vi "Read Sensor Data.vi"(8 "error in (no error)":errorcluster, 10 "wait ms":u32=500, 11 "VISA Refnum in":refnum<visa-resource-name>) -> (0 "error out":errorcluster, 1 "DataOut":T1, 2 "read buffer":string, 3 "VISA Refnum out":refnum<visa-resource-name>, 5 "Data Not Good":bool)   [LabVIEW 2013]
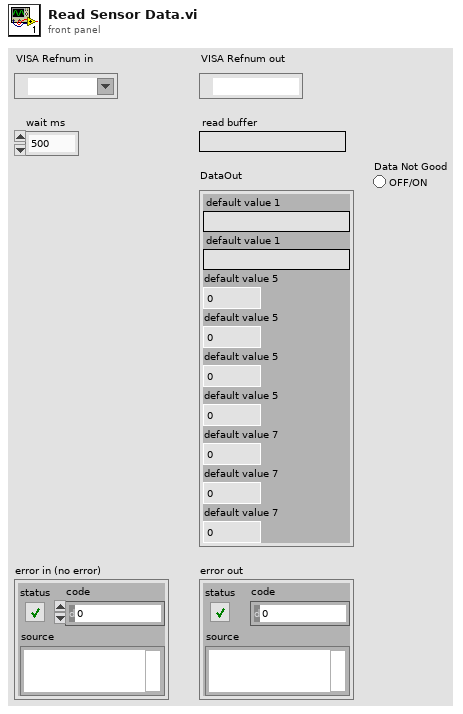
[diagram p1: front panel]
types:
  T1 = cluster{"default value 1":string, "default value 1":string, "default value 5":u32, "default value 5":u32, "default value 5":u32, "default value 5":u32, "default value 7":sgl, "default value 7":sgl, "default value 7":sgl}
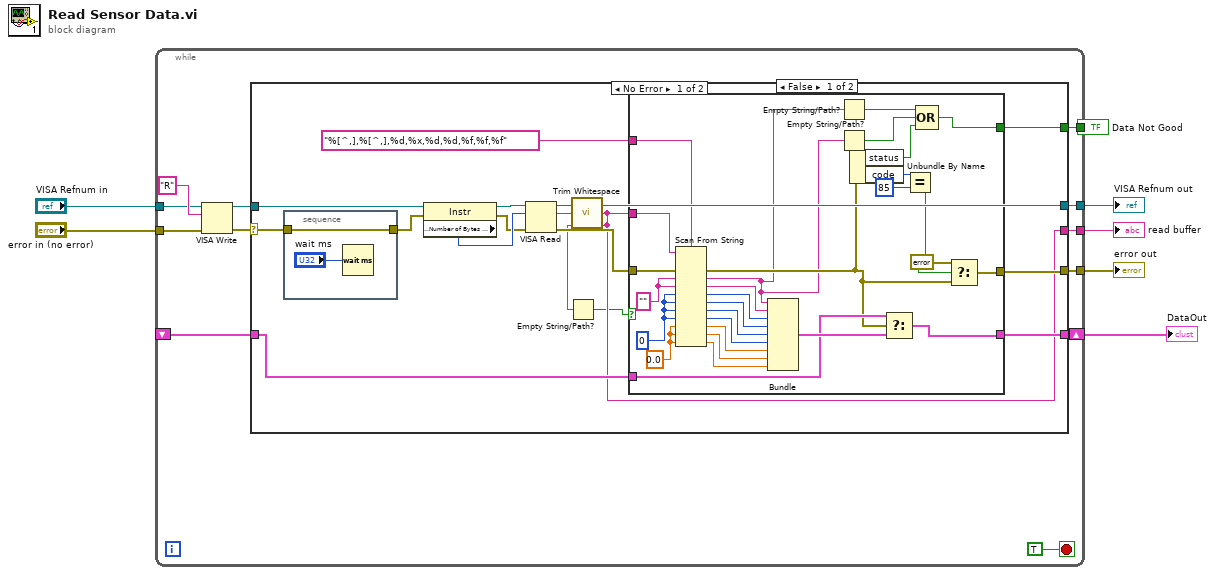
[diagram p0: block diagram]
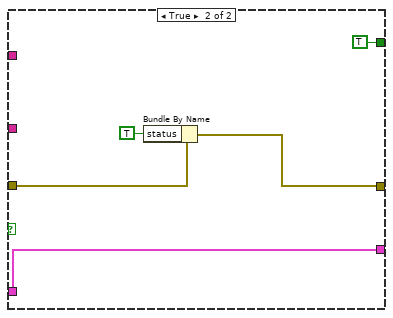
[diagram p2: hidden frame]
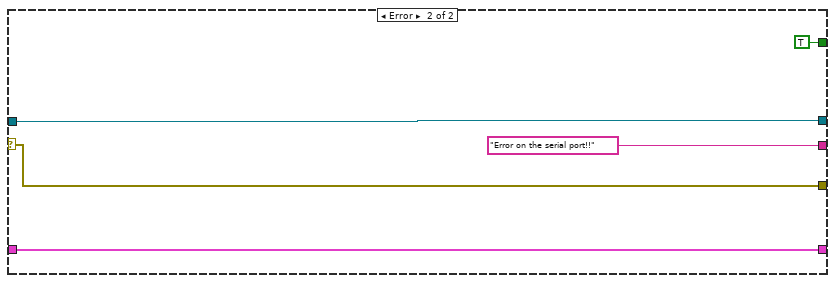
[diagram p3: hidden frame]
diagram:
  n1 = while {
    tunnel: "error in (no error)" -> [w16]
    tunnel: "VISA Refnum in" -> [w15]
    tunnel: [w13] -> w4
    tunnel: [w12] -> w3
    tunnel: [w11] -> w2
    tunnel: [w9] -> w1
    shift-right: [w14] -> w5
    shift-left: _ -> [w10]
    stop <- TRUE stop-if-true
    n2 = VISA Write(VISA resource name=w15, write buffer="R" ("string"), error in (no error)=w16) -> (VISA resource name out=w17:refnum<visa-resource-name>, error out=w18:errorcluster)  [unwired: 1 out]
    n3 = case shown="No Error" w18 {
      selector: w18 -> [w28 w72]
      tunnel: w17 -> [w30 w75]
      tunnel: [w27 w75] -> w11
      tunnel: [w23 w72] -> w12
      tunnel: [w24 w74] -> w14
      tunnel: [w21 "Error on the serial port!!" ("read buffer")] -> w13
      tunnel: w10 -> [w25 w74]
      tunnel: [w22 TRUE] -> w9
      frame No Error {
        n4 = stacked-sequence {
          tunnel: [w69] -> w31
          tunnel: w28 -> [w69]
          frame #0 {
            n5 = Wait (ms)(milliseconds to wait="wait ms") -> ()  [unwired: 1 out]
          }
        }
        n6 = property class="Instr"(reference=w30, error in=w31) -> (reference out=w33:refnum<visa-resource-name>, error out=w32:errorcluster, "Serial Settings:Number of Bytes at Serial Port"=w34:u32)
        n7 = VISA Read(VISA resource name=w33, byte count=w34, error in (no error)=w32) -> (VISA resource name out=w27:refnum<visa-resource-name>, read buffer=w26:string, error out=w29:errorcluster)  [unwired: 1 out]
        n8 = call <vilib>:"Trim Whitespace.vi"("string"=w26) -> ("trimmed string"=w21:string)  [unwired: 1 in]
        n9 = Empty String/Path?(string/path=w21) -> (empty?=w20:bool)
        n10 = case shown="False" w20 {
          tunnel: "%[^,],%[^,],%d,%x,%d,%d,%f,%f,%f" ("String") -> [w63 _]
          tunnel: w29 -> [w51 w65]
          tunnel: w21 -> [w50 _]
          tunnel: w25 -> [w48 w68]
          tunnel: [w47 w68] -> w24
          tunnel: [w41 w64] -> w23
          tunnel: [w36 TRUE] -> w22
          frame False {
            w53 = sgl 0.0 ("default value 7")
            w62 = "" ("default value 1")
            w52 = u32 0 ("default value 5")
            n11 = Scan From String(format string=w63, input string=w50, error in=w51, default 1=w62, default 2=w62, default 3=w52, default 4=w52, default 5=w52, default 6=w52, default 7=w53, default 8=w53, default 9=w53) -> (error out=w43:errorcluster, output 1=w40:string, output 2=w61:string, output 3=w60:u32, output 4=w59:u32, output 5=w58:u32, output 6=w57:u32, output 7=w56:sgl, output 8=w55:sgl, output 9=w54:sgl)  [unwired: 1 in, 2 out]
            n12 = Bundle("default value 1"=w40, "default value 1"=w61, "default value 5"=w60, "default value 5"=w59, "default value 5"=w58, "default value 5"=w57, "default value 7"=w56, "default value 7"=w55, "default value 7"=w54) -> (w49:T1)  [unwired: 1 in]
            n13 = Empty String/Path?(string/path=w40) -> (empty?=w39:bool)
            n14 = Empty String/Path?(string/path=w40) -> (empty?=w38:bool)
            n15 = Unbundle By Name(w43) -> ("status"=w37:bool, "code"=w46:i32)
            n16 = Select(t=w48, s=w43, f=w49) -> (s? t:f=w47:T1)
            n17 = Equal?(x=w46, y=85) -> (x = y?=w44:bool)
            n18 = Compound Arithmetic op=OR(w39, w38, w37) -> (w36:bool)
            n19 = Select(t=errorcluster {"status"=FALSE, "code"=0, "source"=""}, s=w44, f=w43) -> (s? t:f=w41:errorcluster)
          }
          frame True {
            n20 = Bundle By Name(cluster=w65, "status"=TRUE) -> (w64:errorcluster)
          }
        }
      }
      frame Error {
      }
    }
  }
  "DataOut" <- w5
  "read buffer" <- w4
  "error out" <- w3
  "VISA Refnum out" <- w2
  "Data Not Good" <- w1
